vi "rgerge.vi"(11 "Data In":T1) -> (3 "Data Out":T1)   [LabVIEW 2016]
doc: "Assert Component\nAssert Name: rgerge\nData Type: Double Float\nDeveloped by UKHornP\nEvaluation String: X = 453545.000000\nDescription: egerger"
uses:
  LabVIEW Data/Quick Drop Plugins/_CreateNewAssertSupport/Templates/NC Templates/dbl.ctl
  Core/Assert API Components/Failure Actions.ctl
  Core/Assert API Components/Assert API Components.lvlib
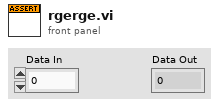
[diagram p1: front panel]
types:
  T1 = typedef "dbl.ctl" = dbl
  T2 = typedef "Assert API Components.lvlib/Failure Actions.ctl" = enum16{"None", "Log To File", "Pause Execution", "Abort Execution"}
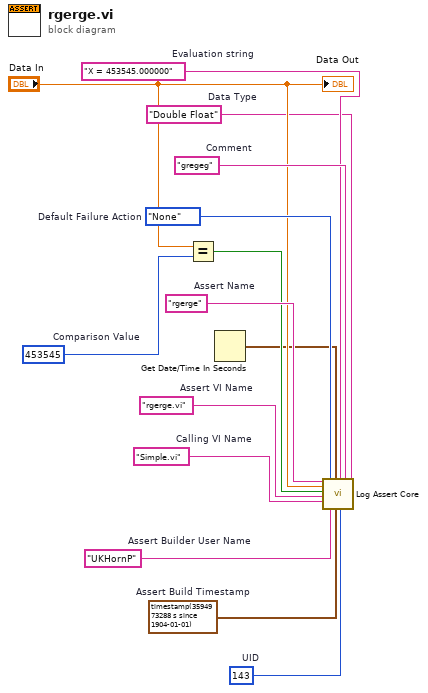
[diagram p0: block diagram]
diagram:
  w1 = 143  # UID
  w3 = "rgerge.vi"  # Assert VI Name
  w4 = "Simple.vi"  # Calling VI Name
  w5 = timestamp(3594973288.311156 s since 1904-01-01)  # Assert Build Timestamp
  w6 = "UKHornP"  # Assert Builder User Name
  w7 = "Double Float"  # Data Type
  w11 = "gregeg"  # Comment
  w8 = "X = 453545.000000"  # Evaluation string
  w13 = Failure_Actions."None"  # Default Failure Action
  w14 = "rgerge"  # Assert Name
  w12 = 453545  # Comparison Value
  n1 = Equal?(x="Data In", y=w12) -> (x = y?=w9:bool)
  n2 = Get Date/Time In Seconds() -> (seconds since 1Jan1904=w2:timestamp)
  n3 = call "Log Assert Core.vi"("Assert Name"=w14, "Data Value"="Data In", "Status"=w9, "Assert VI Name"=w3, "Calling VI Name"=w4, "Failure Action"=w13, "Assert Builder User Name"=w6, "Last Update"=w2, "Assert Build Timestamp"=w5, "Evaluation String"=w8, "Assert VI UID"=w1, "Comment"=w11, "Data Type"=w7) -> ()  [unwired: 7 in]
  "Data Out" <- "Data In"
